vi "Tab_Control.vi"(8 "error in (no error)":errorcluster, 11 "Tab Control":refnum<vi>) -> (0 "error out":errorcluster)   [LabVIEW 2023]
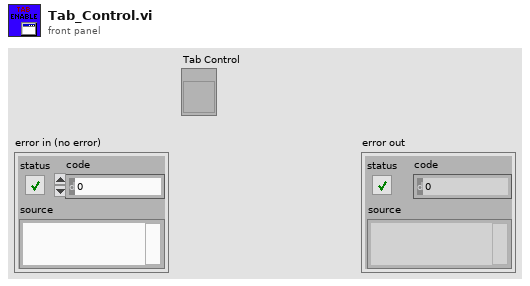
[diagram p1: front panel]
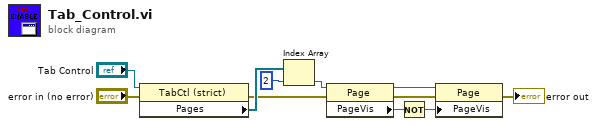
[diagram p0: block diagram]
diagram:
  n1 = property class="TabCtl (strict)"(reference="Tab Control", error in="error in (no error)") -> (error out=w8:errorcluster, "Pages"=w9:refnum<vi>[])  [unwired: 1 out]
  n2 = Index Array(array=w9, index=2) -> (element=w7:refnum<vi>)
  n3 = property class="Page"(reference=w7, error in=w8) -> (reference out=w5:refnum<vi>, error out=w3:errorcluster, "PageVis"=w6:bool)
  n4 = Not(x=w6) -> (.not. x?=w4:bool)
  n5 = property class="Page"(reference=w5, error in=w3, "PageVis"=w4) -> (error out=→"error out":errorcluster)  [unwired: 1 out]
